vi "Clear.vi"(8 "error in (no error)":errorcluster, 11 "Mock Job Handler In":refnum<class "Mock Job Handler.lvclass">) -> (0 "error out":errorcluster)   [LabVIEW 2020, in "Mock Job Handler.lvclass"]
doc: "Clears any resorces allocated during initialization."
uses:
  Mock Job Handler.lvclass
  Mock Job Handler.lvclass/Mock Job Handler.ctl
  <vilib>/Astemes/Triarc Framework/Base/Base.lvclass
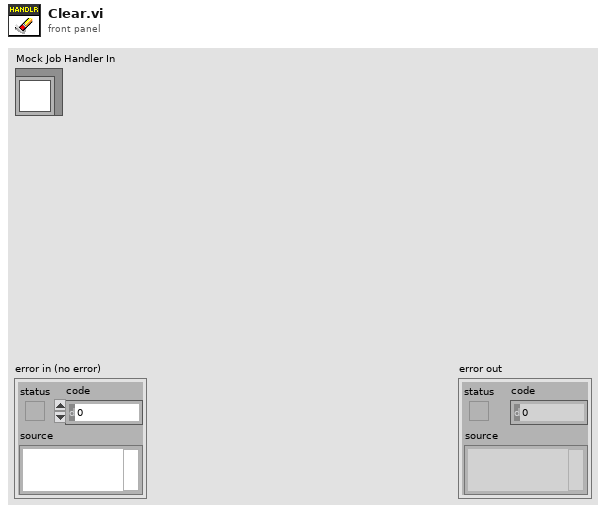
[diagram p1: front panel]
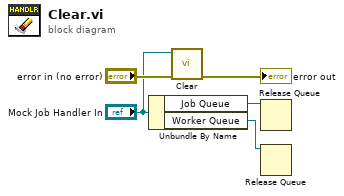
[diagram p0: block diagram]
diagram:
  n1 = Unbundle By Name("Mock Job Handler In") -> ("Job Queue"=w2:refnum<queue>, "Worker Queue"=w1:refnum<queue>)
  n2 = call-parent "Clear.vi"("error in (no error)"="error in (no error)", "Base In"="Mock Job Handler In") -> ("error out"=→"error out":errorcluster)  [unwired: 9 in]
  n3 = Release Queue(queue=w2) -> ()  [unwired: 2 in, 3 out]
  n4 = Release Queue(queue=w1) -> ()  [unwired: 2 in, 3 out]
